vi "T1 VI Template (With Error Terminals).vi"(8 "Error In":errorcluster) -> (0 "Error Out":errorcluster)   [LabVIEW 2016]
doc: "<add documentation here>"
panel:
  # "Development\nControls or indicators that are useful for development or testing, but which are not outputs of the VI."
  # "Input\nInputs to the VI"
  # "Output\nOutputs of the VI"
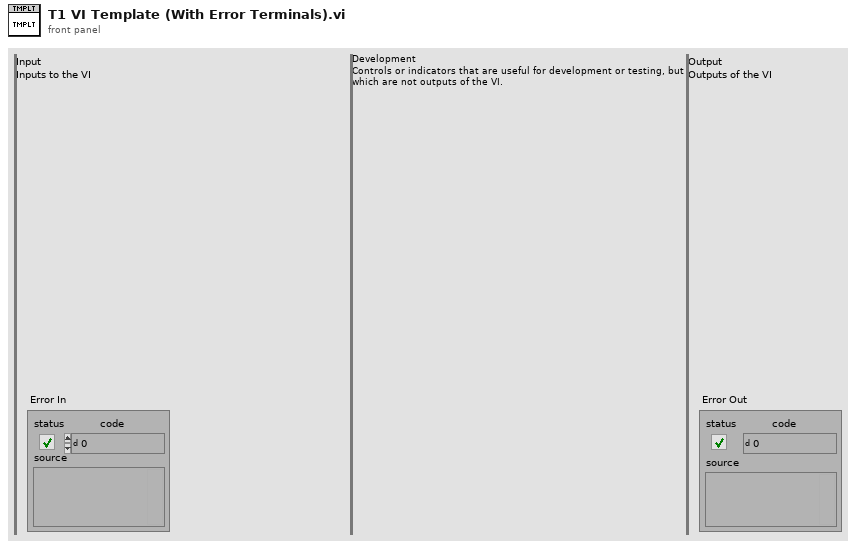
[diagram p1: front panel]
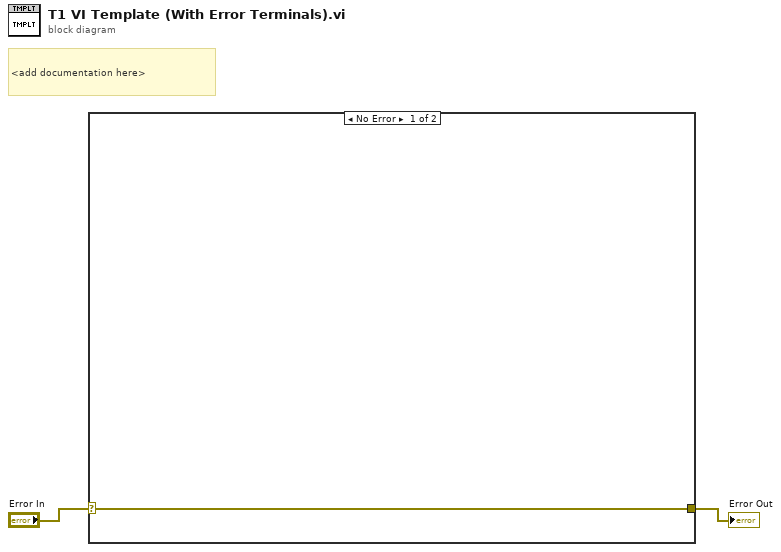
[diagram p0: block diagram]
diagram:
  # "<add documentation here>"
  n1 = case shown="No Error" "Error In" {
    selector: "Error In" -> [w3 w4]
    tunnel: [w3 w4] -> w1
    frame No Error {
    }
    frame Error {
    }
  }
  "Error Out" <- w1
